vi "Check Hardware In.vi"(8 "error in (no error)":errorcluster, 10 "Hardware Name":string, 11 "Controller in":refnum<class "Controller.lvclass">) -> (0 "error out":errorcluster, 3 "Controller out":refnum<class "Controller.lvclass">)   [LabVIEW 2015, in "Controller Actor.lvlib" / "Controller.lvclass"]
uses:
  Controller.lvclass
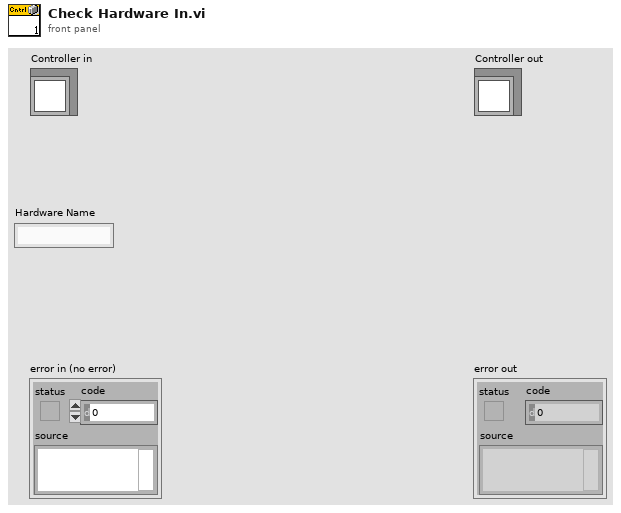
[diagram p1: front panel]
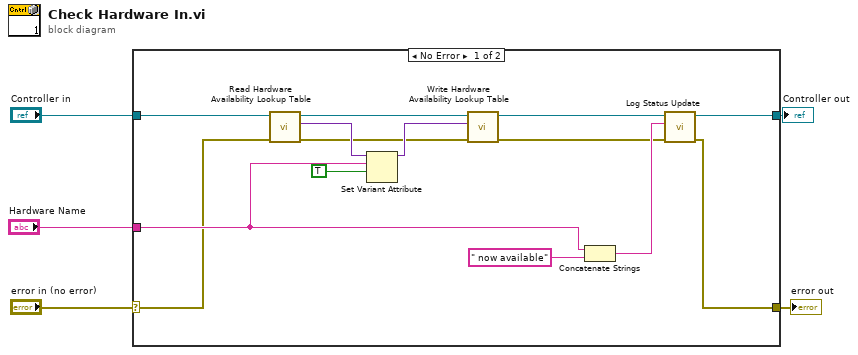
[diagram p0: block diagram]
diagram:
  n1 = case shown="No Error" "error in (no error)" {
    selector: "error in (no error)" -> [w7 w21]
    tunnel: [w6 w21] -> w4
    tunnel: [w10 w20] -> w2
    tunnel: "Controller in" -> [w19 w20]
    tunnel: "Hardware Name" -> [w14 _]
    frame No Error {
      n2 = call "Read Hardware Availability Lookup Table.vi"("error in (no error)"=w7, "Controller in"=w19) -> ("error out"=w9:errorcluster, "Hardware Availability Lookup Table"=w17:variant, "Controller out"=w18:refnum<class "Controller.lvclass">)  [unwired: 7 in]
      n3 = Set Variant Attribute(Variant=w17, name=w14, value=TRUE) -> (Variant out=w16:variant)  [unwired: 1 in, 2 out]
      n4 = call "Write Hardware Availability Lookup Table.vi"("error in (no error)"=w9, "Hardware Availability Lookup Table"=w16, "Controller in"=w18) -> ("error out"=w8:errorcluster, "Controller out"=w11:refnum<class "Controller.lvclass">)  [unwired: 7 in]
      n5 = Concatenate Strings(w14, " now available" ("string")) -> (w12:string)
      n6 = call-dynamic "Log Status Update.vi"("error in (no error)"=w8, "String"=w12, "Controller in"=w11) -> ("error out"=w6:errorcluster, "Controller out"=w10:refnum<class "Controller.lvclass">)  [unwired: 7 in]
    }
    frame Error {
    }
  }
  "error out" <- w4
  "Controller out" <- w2
